vi "Valhalla RS232 Initialize.vi"(5 "Baud Rate":u32=115200, 6 "Flow Control":u16(ring) items=["None", "XON/XOFF", "RTS/CTS", "XON/XOFF & RTS/CTS", "DTR/DSR", "XON/XOFF & DTR/DSR"], 7 "Data Bits":u16=8, 8 "error in (no error)":errorcluster, 9 "Stop Bits":u16(ring)=10 items=["1.0"=10, "1.5"=15, "2.0"=20], 10 "Parity":u16(ring) items=["None", "Odd", "Even", "Mark", "Space"], 11 "VISA Refnum in":refnum<visa-resource-name>) -> (0 "error out":errorcluster, 3 "VISA Refnum out":refnum<visa-resource-name>)   [LabVIEW 2018]
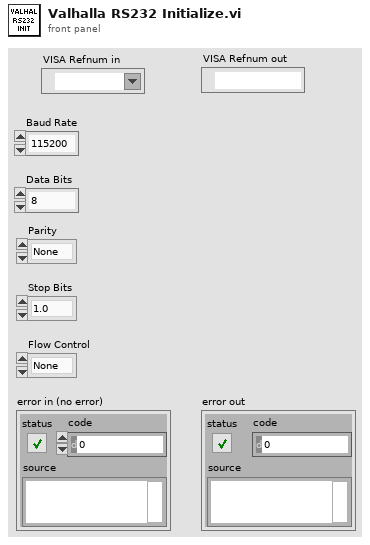
[diagram p1: front panel]
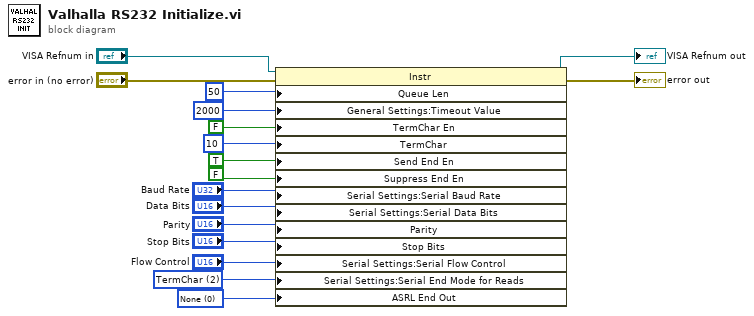
[diagram p0: block diagram]
diagram:
  w13 = u16 0 items=["None", "Last Bit", "TermChar", "Break"] ("Serial Settings:End Mode for Writes")
  w12 = u16 2 items=["None", "Last Bit", "TermChar"] ("Serial Settings:End Mode for Reads")
  n1 = property class="Instr"(reference="VISA Refnum in", error in="error in (no error)", "Queue Len"=u32 50 ("General Settings:Maximum Queue Length"), "General Settings:Timeout Value"=u32 2000, "TermChar En"=FALSE ("Message Based Settings:Termination Character Enable"), "TermChar"=u8 10 ("Message Based Settings:Termination Character"), "Send End En"=TRUE ("Message Based Settings:Send End Enable"), "Suppress End En"=FALSE ("Message Based Settings:Suppress End Enable"), "Serial Settings:Serial Baud Rate"="Baud Rate", "Serial Settings:Serial Data Bits"="Data Bits", "Parity"="Parity", "Stop Bits"="Stop Bits", "Serial Settings:Serial Flow Control"="Flow Control", "Serial Settings:Serial End Mode for Reads"=w12, "ASRL End Out"=w13) -> (reference out=→"VISA Refnum out":refnum<visa-resource-name>, error out=→"error out":errorcluster)
